vi "get_notDeleted.vi"(0 "HGF_SVVarManVisitor_delete":refnum<class "HGF_SVVarManVisitor_delete.lvclass">, 5 "error in (no error)":errorcluster) -> (14 "dup HGF_SVVarManVisitor_delete":refnum<class "HGF_SVVarManVisitor_delete.lvclass">, 16 "not deleted?":bool, 19 "error out":errorcluster)   [LabVIEW 2012, in "HGF_SV.lvlib" / "HGF_SVVarManVisitor_delete.lvclass"]
uses:
  HGF_SVVarManVisitor_delete.lvclass
  HGF_SVVarManVisitor_delete.lvclass/HGF_SVVarManVisitor_delete.ctl
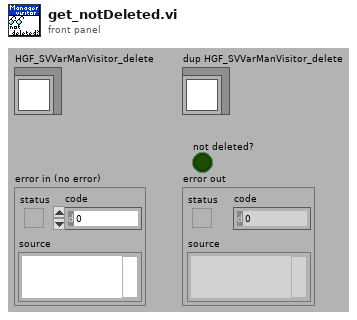
[diagram p1: front panel]
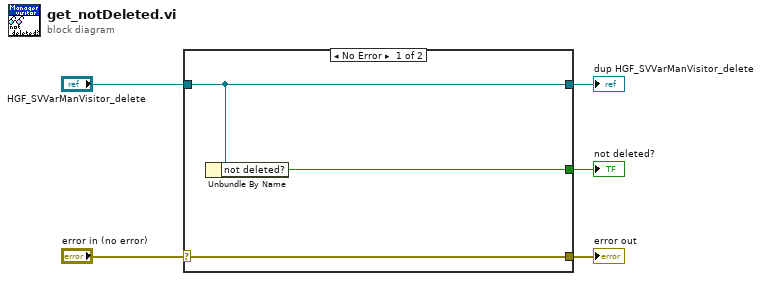
[diagram p0: block diagram]
diagram:
  n1 = case shown="No Error" "error in (no error)" {
    selector: "error in (no error)" -> [w8 w9]
    tunnel: [w8 w9] -> w4
    tunnel: [w7 w10] -> w2
    tunnel: "HGF_SVVarManVisitor_delete" -> [w7 w10]
    tunnel: [w6 _] -> w1
    frame No Error {
      n2 = Unbundle By Name(w7) -> ("not deleted?"=w6:bool)
    }
    frame Error {
    }
  }
  "error out" <- w4
  "dup HGF_SVVarManVisitor_delete" <- w2
  "not deleted?" <- w1
